vi "Calculate Chi-CO2.vi"(0 "Chi_CO2_A":dbl format="%#_13g", 1 "z_i":dbl format="%#_13g", 2 "z_t":dbl format="%#_13g", 3 "z_m":dbl format="%#_13g", 5 "Chi_H2O_A":dbl format="%#_13g", 7 "Chi_H2O_B":dbl format="%#_13g", 9 "Raw_CO2_A":dbl format="%#_13g", 11 "Raw_CO2_B":dbl format="%#_13g", 12 "T [C]":dbl format="%#_13g", 13 "P [kPa]":dbl format="%#_13g", 14 "S":dbl=1.39327 format="%#_13g") -> (8 "Chi_CO2_B":dbl)   [LabVIEW 2010]
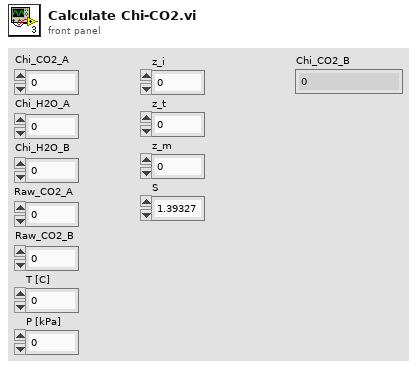
[diagram p1: front panel]
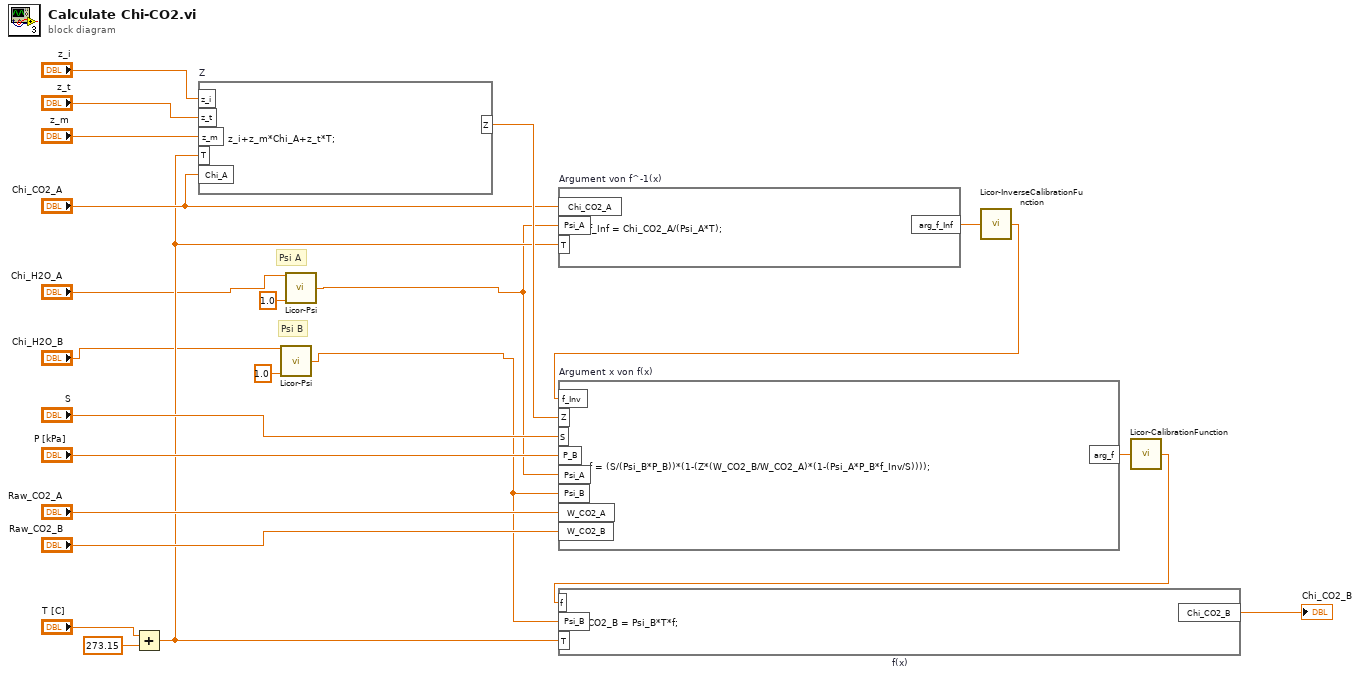
[diagram p0: block diagram]
diagram:
  # "Psi A"
  # "Psi B"
  n1 = Add(x="T [C]", y=273.15) -> (x+y=w11:dbl)
  n2 = formula code="Z = z_i+z_m*Chi_A+z_t*T;"("z_i"="z_i", "z_t"="z_t", "z_m"="z_m", "T"=w11, "Chi_A"="Chi_CO2_A") -> ("Z"=w21:dbl)
  n3 = call "Licor-Psi.vi"("Chi_i"="Chi_H2O_B", "a"=1.0) -> ("Psi_i"=w9:dbl)  [unwired: 13 in]
  n4 = call "Licor-Psi.vi"("Chi_i"="Chi_H2O_A", "a"=1.0) -> ("Psi_i"=w10:dbl)  [unwired: 13 in]
  n5 = formula code="arg_f_Inf = Chi_CO2_A/(Psi_A*T);" "Argument von f^-1(x)"("Chi_CO2_A"="Chi_CO2_A", "Psi_A"=w10, "T"=w11) -> ("arg_f_Inf"=w8:dbl)
  n6 = call "Licor-InverseCalibrationFunction.vi"("x"=w8) -> ("f_Inv(x)"=w7:dbl)  [unwired: 14 in]
  n7 = formula code="arg_f = (S/(Psi_B*P_B))*(1-(Z*(W_CO2_B/W_CO2_A)*(1-(Psi_A*P_B*f_Inv/S))));" "Argument x von f(x)"("f_Inv"=w7, "Z"=w21, "S"="S", "P_B"="P [kPa]", "Psi_A"=w10, "Psi_B"=w9, "W_CO2_A"="Raw_CO2_A", "W_CO2_B"="Raw_CO2_B") -> ("arg_f"=w6:dbl)
  n8 = call "Licor-CalibrationFunction.vi"("x"=w6) -> ("f(x)"=w5:dbl)  [unwired: 14 in]
  n9 = formula code="Chi_CO2_B = Psi_B*T*f;" "f(x)"("f"=w5, "Psi_B"=w9, "T"=w11) -> ("Chi_CO2_B"=→"Chi_CO2_B":dbl)
